vi "Test Progress.vi"(8 "error in (no error)":errorcluster, 9 "Current State":string, 10 "Test Name":string, 11 "Test Application Controller in":refnum<class "Test Application Controller.lvclass">) -> (0 "error out":errorcluster, 3 "Test Application Controller out":refnum<class "Test Application Controller.lvclass">)   [LabVIEW 2017, in "Test Application Controller.lvlib" / "Test Application Controller.lvclass"]
uses:
  Test Application Controller.lvclass
  C:/Program Files (x86)/National Instruments/LabVIEW 2017/vi.lib/ActorFramework/Actor/Actor.lvclass
  Test Application Controller.lvclass/Test Application Controller.ctl
  User Interface Messages/Update Progress Msg/Update Progress Msg.lvclass/Update Progress Msg.ctl
  <vilib>/ActorFramework/Message Enqueuer/Message Enqueuer.lvclass/Message Enqueuer.ctl
  <vilib>/ActorFramework/Actor/Actor.lvclass/Actor.ctl
  Test Application Controller Messages/Launch Test Msg/Launch Test Msg.lvclass/Launch Test Msg.ctl
  <vilib>/ActorFramework/Message Enqueuer/Enqueue.vi
  <vilib>/ActorFramework/Message Enqueuer/Init from Existing Queue.vi
  User Interface Messages/Update Progress Msg/Update Progress Msg.lvclass
  C:/Program Files (x86)/National Instruments/LabVIEW 2017/vi.lib/ActorFramework/Message/Message.lvclass
  Test Application Controller Messages/Launch Test Msg/Launch Test Msg.lvclass
  <vilib>/ActorFramework/Message Priority Queue/Priority Enqueue.vi
  <vilib>/ActorFramework/Message Enqueuer/Message Enqueuer.lvclass
  <vilib>/ActorFramework/Actor/Actor.lvclass
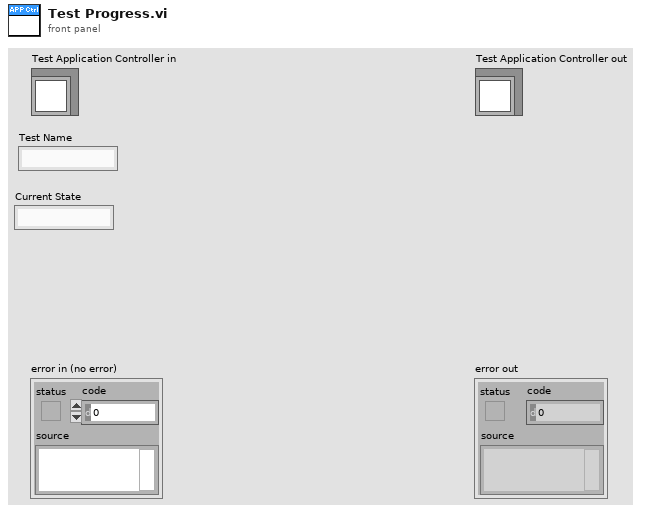
[diagram p1: front panel]
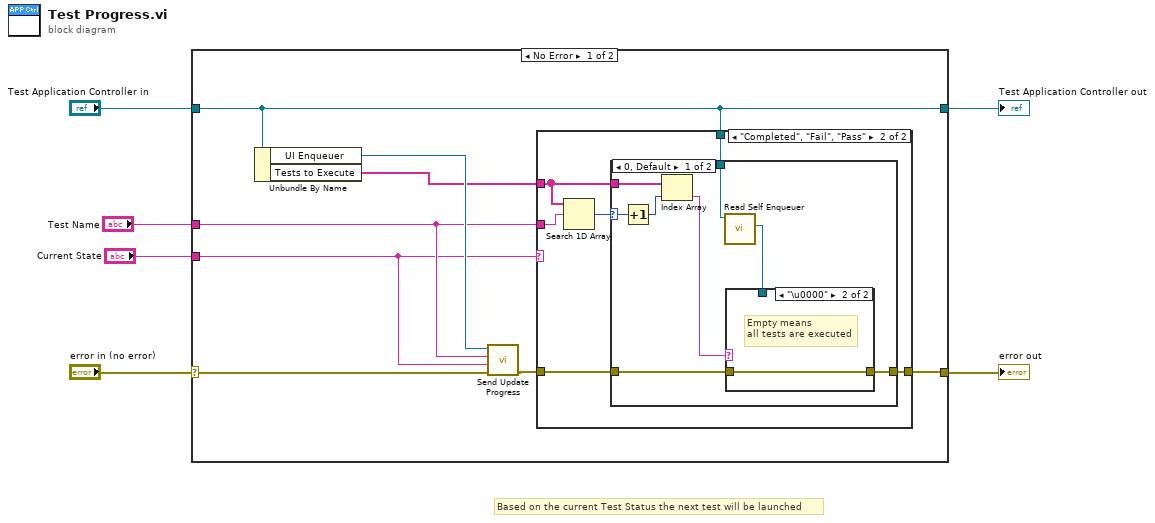
[diagram p0: block diagram]
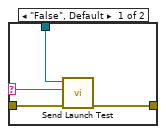
[diagram p3: hidden frame]
diagram:
  # "Based on the current Test Status the next test will be launched"
  n1 = case shown="No Error" "error in (no error)" {
    selector: "error in (no error)" -> [w13 w37]
    tunnel: [w9 w37] -> w5
    tunnel: [w7 w36] -> w3
    tunnel: "Test Application Controller in" -> [w7 w36]
    tunnel: "Test Name" -> [w11 _]
    tunnel: "Current State" -> [w8 _]
    frame No Error {
      n2 = Unbundle By Name(w7) -> ("UI Enqueuer"=w14:refnum<class "Message Enqueuer.lvclass">, "Tests to Execute"=w12:string[])
      n3 = call "Send Update Progress.vi"("error in (no error)"=w13, "Current State"=w8, "Test Name"=w11, "Message Enqueuer"=w14) -> ("error out"=w10:errorcluster)  [unwired: 6 in, 1 out]
      n4 = case shown="\"Completed\", \"Fail\", \"Pass\"" w8 {
        tunnel: w12 -> [_ w20]
        tunnel: w11 -> [_ w21]
        tunnel: w10 -> [w15 w19]
        tunnel: [w15 w18] -> w9
        tunnel: w7 -> [_ w17]
        frame "False", Default {
        }
        frame "Completed", "Fail", "Pass" {
          n5 = Search 1D Array(1D array=w20, element=w21) -> (index of element=w16:i32)  [unwired: 1 in]
          n6 = case shown="0, Default" w16 {
            selector: w16 -> [w22 _]
            tunnel: w20 -> [w29 _]
            tunnel: w19 -> [w28 w35]
            tunnel: [w27 w35] -> w18
            tunnel: w17 -> [w26 _]
            frame 0, Default {
              n7 = Increment(x=w22) -> (x+1=w24:i32)
              n8 = Index Array(array=w29, index=w24) -> (element=w23:string)
              n9 = call <vilib>:"Read Self Enqueuer.vi"("Actor"=w26) -> ("Self Enqueuer"=w25:refnum<class "Message Enqueuer.lvclass">)  [unwired: 10 in]
              n10 = case shown="\"\"" w23 {
                selector: w23 -> [w30 _]
                tunnel: w28 -> [w33 w34]
                tunnel: [w32 w34] -> w27
                tunnel: w25 -> [w31 _]
                frame "False", Default {
                  n11 = call "Send Launch Test.vi"("error in (no error)"=w33, "Test Name"=w30, "Message Enqueuer"=w31) -> ("error out"=w32:errorcluster)  [unwired: 7 in, 1 out]
                }
                frame "\u0000" {
                  # "Empty means \nall tests are executed"
                }
              }
            }
            frame -1 {
            }
          }
        }
      }
    }
    frame Error {
    }
  }
  "error out" <- w5
  "Test Application Controller out" <- w3
